vi "Intrumento_2.vi"() -> ()   [LabVIEW 2016]
uses:
  Global_2.vi
  Global_1.vi
panel:
  out "Numeric Control_1":dbl
  out "Boolean_1":bool
  in  "Numeric Control_2":dbl
  in  "Boolean_2":bool
  in  "Stop Button":bool
  out "Usuario 1":string
  in  "Usuario 2":string
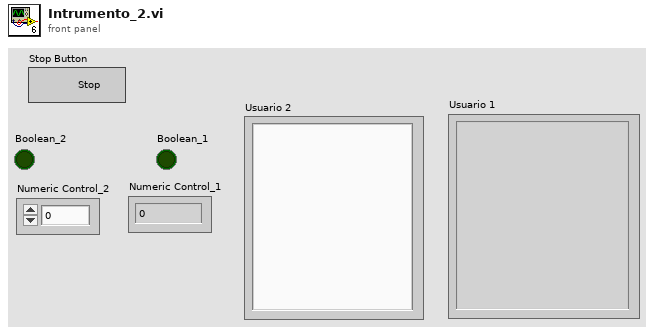
[diagram p1: front panel]
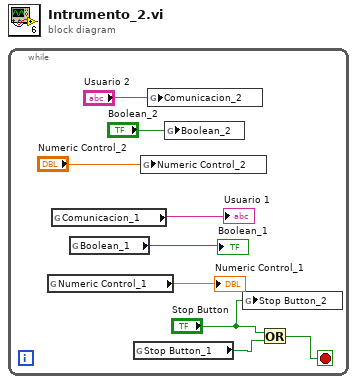
[diagram p0: block diagram]
diagram:
  n1 = while {
    stop <- w2 stop-if-true
    n2 = global read "Global_1.vi" "Numeric Control_1"() -> (→"Numeric Control_1":dbl)
    n3 = global read "Global_1.vi" "Comunicacion_1"() -> (→"Usuario 1":string)
    n4 = global read "Global_1.vi" "Boolean_1"() -> (→"Boolean_1":bool)
    n5 = global read "Global_1.vi" "Stop Button_1"() -> (w3:bool)
    n6 = global write "Global_2.vi" "Numeric Control_2"("Numeric Control_2") -> ()
    n7 = global write "Global_2.vi" "Comunicacion_2"("Usuario 2") -> ()
    n8 = global write "Global_2.vi" "Boolean_2"("Boolean_2") -> ()
    n9 = global write "Global_2.vi" "Stop Button_2"("Stop Button") -> ()
    n10 = Or(x="Stop Button", y=w3) -> (x .or. y?=w2:bool)
  }
